vi "Interface_Dispatch_Initialize Module.vi"(8 "error in (no error)":errorcluster, 11 "Interface_Dispatch in":refnum<class "Interface_Dispatch.lvclass">) -> (0 "error out":errorcluster, 1 "Dependencies":T1, 2 "TagDescriptions":refnum<class "tag descriptor.lvclass">[](array[class]), 3 "Interface_Dispatch out":refnum<class "Interface_Dispatch.lvclass">)   [LabVIEW 2015, in "Interface_Dispatch.lvclass"]
uses:
  Interface_Dispatch.lvclass
  <vilib>/NI/Tag Bus/tag/tag descriptor.lvclass
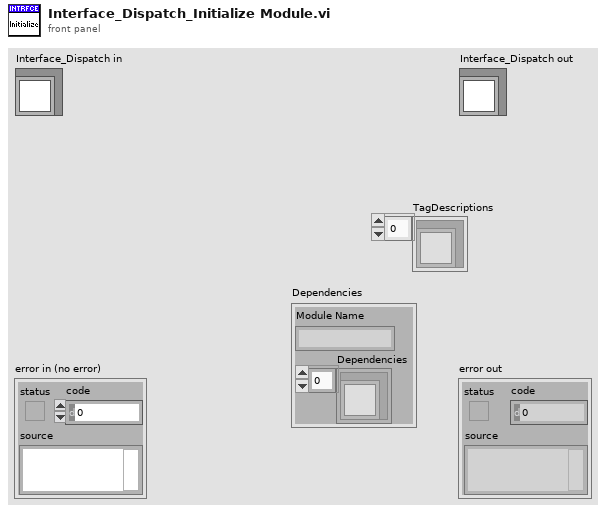
[diagram p1: front panel]
types:
  T1 = cluster{"Module Name":string, "Dependencies":refnum<class "tag descriptor.lvclass">[]}
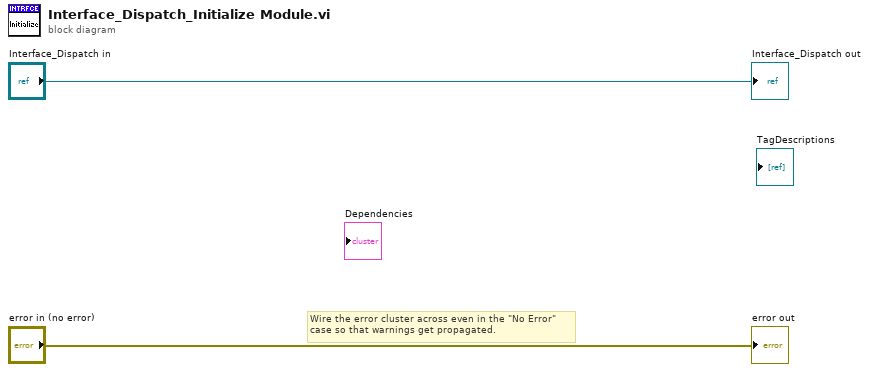
[diagram p0: block diagram]
diagram:
  # "Wire the error cluster across even in the \"No Error\"\ncase so that warnings get propagated."
  "error out" <- "error in (no error)"
  "Interface_Dispatch out" <- "Interface_Dispatch in"
